vi "Saved example data.vi"() -> ()   [LabVIEW 2017]
uses:
  Scripting Examples/SubVIs/Routing Channel Configuration.ctl
  Scripting Examples/SLSC Switch Examples.lvlib
panel:
  in  "Channel Configurations":T1[](array[typedef])=[{"Channel Name"="Window Up", "Initial State"="No Connections", "Description"="Window-Up Sensor State", "State Configurations"=[{"Name"="No Connections", "Description"="no connections", "Value"=-1.0, "Connection List"=[]}, {"Name"="Passthrough", "Description"="sensor connected", "Value"=1.0, "Connection List"=[{"Resource"="SLSC-12001-0317E1AA-Mod2", "Source"="DUT_Ch0", "Destination"="LOAD_Ch0"}]}, {"Name"="Short to Ground", "Description"="sensor faulted to ground", "Value"=2.0, "Connection List"=[{"Resource"="SLSC-12001-0317E1AA-Mod2", "Source"="DUT_Ch0", "Destination"="BusA"}]}, {"Name"="Short to Power", "Description"="sensor faulted to power", "Value"=3.0, "Connection List"=[{"Resource"="SLSC-12001-0317E1AA-Mod2", "Source"="DUT_Ch0", "Destination"="BusB"}]}, {"Name"="Open Circuit", "Description"="open circuit - not connected", "Value"=4.0, "Connection List"=[]}]}, {"Channel Name"="Window Down", "Initial State"="No Connections", "Description"="Window-Up Sensor State", "State Configurations"=[{"Name"="No Connections", "Description"="no connections", "Value"=-1.0, "Connection List"=[]}, {"Name"="Passthrough", "Description"="sensor connected", "Value"=1.0, "Connection List"=[{"Resource"="SLSC-12001-0317E1AA-Mod2", "Source"="DUT_Ch1", "Destination"="LOAD_Ch1"}]}, {"Name"="Short to Ground", "Description"="sensor faulted to ground", "Value"=2.0, "Connection List"=[{"Resource"="SLSC-12001-0317E1AA-Mod2", "Source"="DUT_Ch1", "Destination"="BusA"}]}, {"Name"="Short to Power", "Description"="sensor faulted to power", "Value"=3.0, "Connection List"=[{"Resource"="SLSC-12001-0317E1AA-Mod2", "Source"="DUT_Ch1", "Destination"="BusB"}]}, {"Name"="Open Circuit", "Description"="open circuit - not connected", "Value"=4.0, "Connection List"=[]}]}, {"Channel Name"="Two Switches", "Initial State"="No Connections", "Description"="", "State Configurations"=[{"Name"="No Connections", "Description"="", "Value"=-1.0, "Connection List"=[]}, {"Name"="Passthrough", "Description"="passthrough (2 switches)", "Value"=1.0, "Connection List"=[{"Resource"="SLSC-12001-0317E1AA-Mod2", "Source"="DUT_Ch0", "Destination"="LOAD_Ch0"}, {"Resource"="SLSC-12001-0317E1AA-Mod3", "Source"="DUT_Ch0", "Destination"="LOAD_Ch0"}]}, {"Name"="Fault to Ground", "Description"="ground (2 switches)", "Value"=2.0, "Connection List"=[{"Resource"="SLSC-12001-0317E1AA-Mod2", "Source"="DUT_Ch0", "Destination"="BusA"}, {"Resource"="SLSC-12001-0317E1AA-Mod3", "Source"="DUT_Ch0", "Destination"="BusA"}]}, {"Name"="Fault to 12V", "Description"="12V (2 switehes)", "Value"=3.0, "Connection List"=[{"Resource"="SLSC-12001-0317E1AA-Mod2", "Source"="DUT_Ch0", "Destination"="BusB"}, {"Resource"="SLSC-12001-0317E1AA-Mod3", "Source"="DUT_Ch0", "Destination"="BusB"}]}]}]
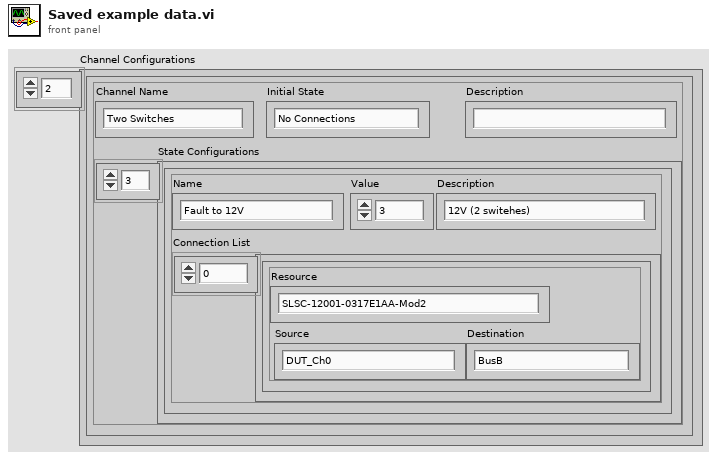
[diagram p1: front panel]
types:
  T1 = typedef "SLSC Switch Examples.lvlib/Routing Channel Configuration.ctl" = cluster{"Channel Name":string, "Initial State":string, "Description":string, "State Configurations":cluster{"Name":string, "Description":string, "Value":dbl, "Connection List":cluster{"Resource":string, "Source":string, "Destination":string}[]}[]}
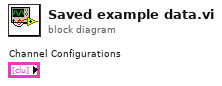
[diagram p0: block diagram]
diagram:
